vi "bin_folder_write.vi"(8 "error in (no error)":errorcluster, 10 "bin_folder":path, 11 "lv-builder in":refnum<class "lv-builder.lvclass">) -> (0 "error out":errorcluster, 3 "lv-builder out":refnum<class "lv-builder.lvclass">)   [LabVIEW 2015, in "lv-builder.lvclass"]
uses:
  lv-builder.lvclass
  lv-builder.lvclass/lv-builder.ctl
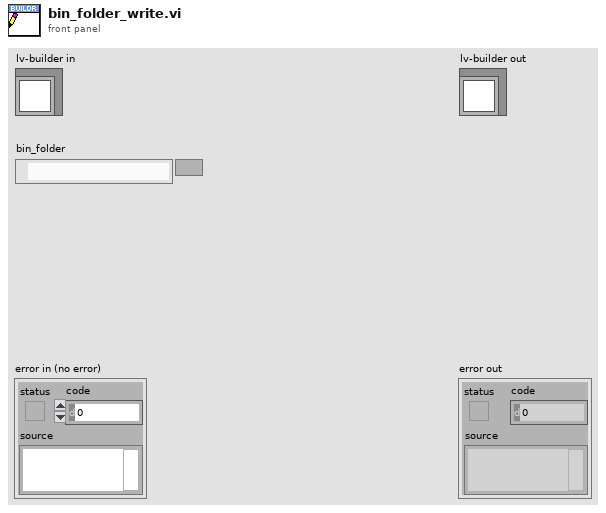
[diagram p1: front panel]
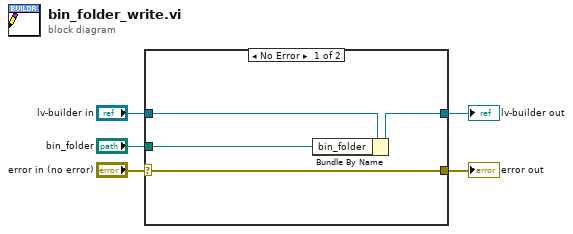
[diagram p0: block diagram]
diagram:
  n1 = case shown="No Error" "error in (no error)" {
    selector: "error in (no error)" -> [w6 w10]
    tunnel: [w6 w10] -> w4
    tunnel: [w8 w11] -> w2
    tunnel: "lv-builder in" -> [w9 w11]
    tunnel: "bin_folder" -> [w7 _]
    frame No Error {
      n2 = Bundle By Name(cluster=w9, "bin_folder"=w7) -> (w8:refnum<class "lv-builder.lvclass">)
    }
    frame Error {
    }
  }
  "error out" <- w4
  "lv-builder out" <- w2
